vi "Timing_DAQ.vi"() -> ()   [LabVIEW 2022 SP3]
uses:
  <vilib>/DAQmx/read.llb/DAQmx Read (Analog 1D DBL NChan 1Samp).vi
  <vilib>/Utility/file.llb/Write Delimited Spreadsheet (string).vi
  <vilib>/DAQmx/configure/timing.llb/DAQmx Timing (Sample Clock).vi
  <vilib>/DAQmx/miscellaneous.llb/DAQmx Fill In Error Info.vi
  <vilib>/Utility/file.llb/Write Delimited Spreadsheet (DBL).vi
panel:
  in  "file path (dialog if empty)":path
  out "iterations":i32
  out "relative seconds":dbl format="%_19f"
  out "eLASPSED time":dbl
  out "data":dbl[](array[numeric]) format="%0.2f"
  out "Gauge":dbl(knob) scale=-11.0..10.0
  out "error out 2":errorcluster
  in  "stop":bool
  in  "rate":dbl=1000.0 format="%0.2f"
  in  "number of samples":i32=100
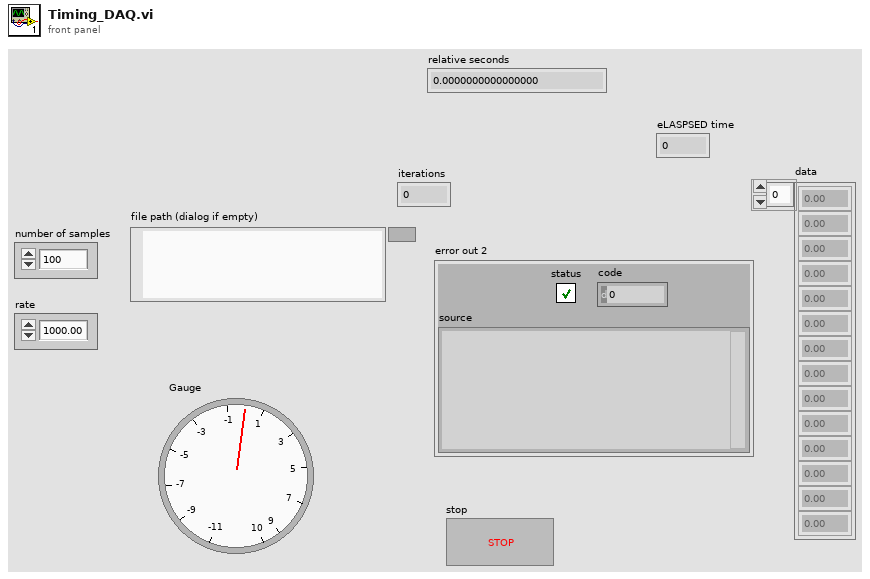
[diagram p1: front panel]
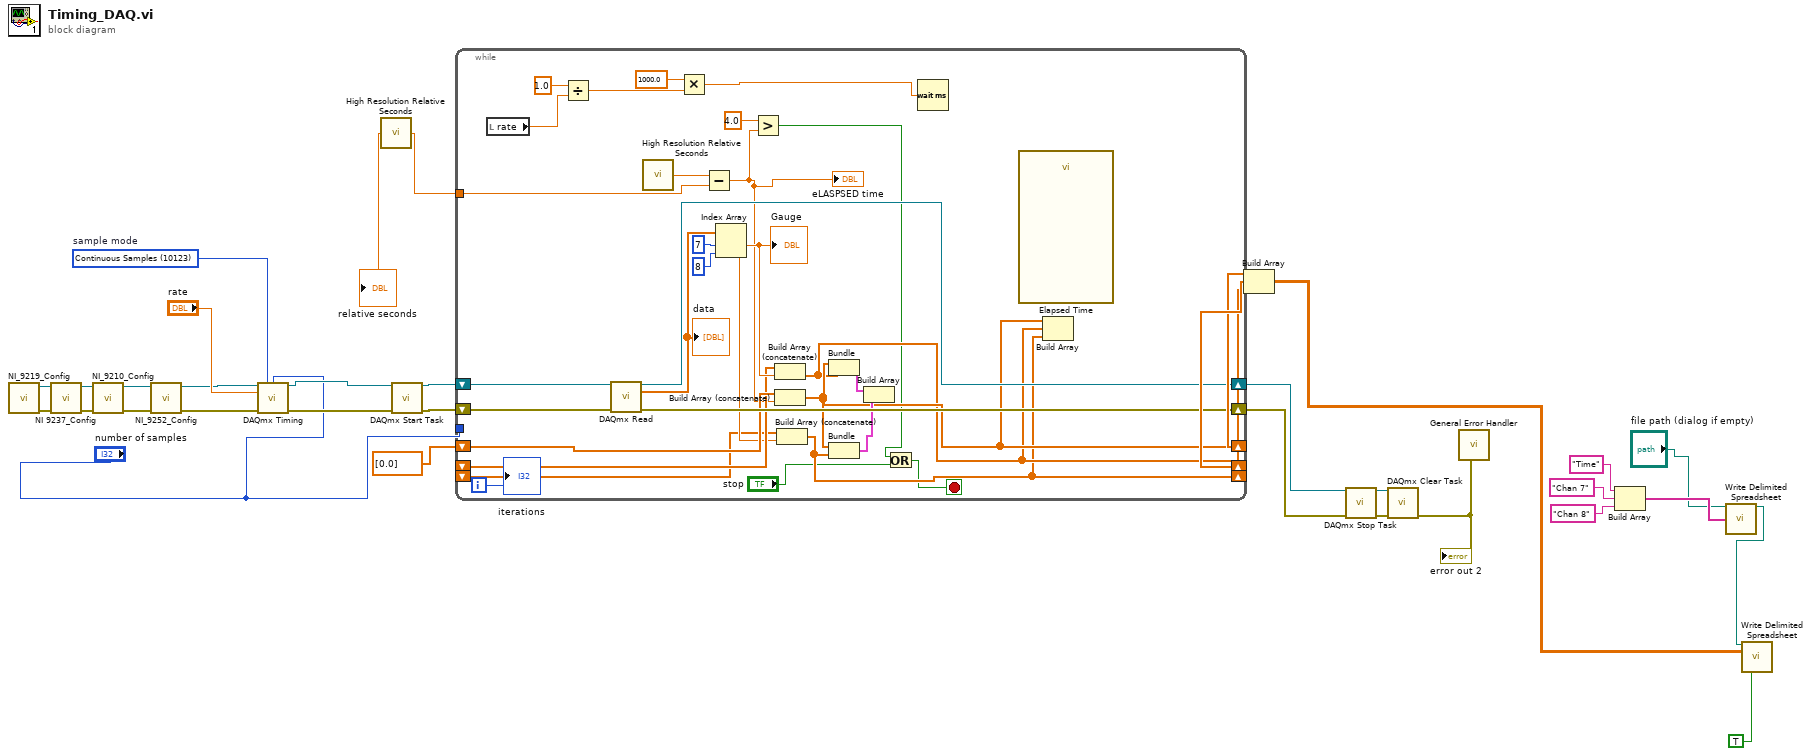
[diagram p0: block diagram]
diagram:
  w27 = 10123 items=["Finite Samples"=10178, "Continuous Samples"=10123, "Hardware Timed Single Point"=12522]  # sample mode
  n1 = call "NI_9219_Config.vi"() -> ("error out"=w28:errorcluster, "task out"=w33:refnum<k21>)  [unwired: 10 in]
  n2 = call "NI 9237_Config.vi"("error in"=w28, "task in"=w33) -> ("error out"=w31:errorcluster, "task out"=w32:refnum<k21>)  [unwired: 8 in]
  n3 = call "NI_9210_Config.vi"("error in"=w31, "task in"=w32) -> ("error out"=w29:errorcluster, "task out"=w30:refnum<k21>)  [unwired: 8 in]
  n4 = call "NI_9252_Config.vi"("error in"=w29, "task in"=w30) -> ("error out"=w24:errorcluster, "task out"=w25:refnum<k21>)  [unwired: 8 in]
  n5 = call-poly <vilib>:"DAQmx Timing.vi"("task/channels in"=w25, "sample mode"=w27, "samples per channel"="number of samples", "rate"="rate", "error in"=w24) -> ("task out"=w3:refnum<k21>, "error out"=w2:errorcluster)  [unwired: 9 in]
  n6 = call <vilib>:"High Resolution Relative Seconds.vi"() -> ("relative seconds"=w17:dbl)
  "relative seconds" <- w17
  n7 = call <vilib>:"DAQmx Start Task.vi"("task/channels in"=w3, "error in"=w2) -> ("task out"=w23:refnum<k21>, "error out"=w22:errorcluster)  [unwired: 12 in]
  n8 = while {
    shift-right: [w61] -> w18
    shift-left: w23 -> [w63]
    shift-right: [w60] -> w19
    shift-left: w22 -> [w62]
    tunnel: "number of samples" -> [_]
    tunnel: w17 -> [w57]
    shift-right: [w46] -> w13
    shift-left: dbl[] [0.0] -> [w56]
    shift-right: [w45] -> w15
    shift-left: _ -> [w53]
    shift-right: [w44] -> w14
    shift-left: _ -> [w50]
    i -> [w47]
    stop <- w42 stop-if-true
    n9 = local read "rate"() -> (w40:dbl)
    n10 = Divide(x=1.0, y=w40) -> (x/y=w39:dbl)
    n11 = call-poly <vilib>:"DAQmx Read.vi"("task/channels in"=w63, "error in"=w62) -> ("task out"=w61:refnum<k21>, "data"=w58:dbl[], "error out"=w60:errorcluster)  [unwired: 11 in]
    "data" <- w58
    n12 = call <vilib>:"High Resolution Relative Seconds.vi"() -> ("relative seconds"=w55:dbl)
    n13 = Multiply(x=1000.0, y=w39) -> (x*y=w37:dbl)
    n14 = Subtract(x=w55, y=w57) -> (x-y=w35:dbl)
    "eLASPSED time" <- w35
    n15 = Index Array(array=w58, index #1=7 ("index"), index #2=8 ("index")) -> (element #1=w54:dbl, element #2=w51:dbl)
    "Gauge" <- w54
    n16 = Greater?(x=4.0, y=w35) -> (0:w34:bool)
    n17 = Build Array (concatenate)(w53, w54) -> (w45:dbl[])
    n18 = Build Array (concatenate)(w56, w35) -> (w46:dbl[])
    n19 = Build Array (concatenate)(w50, w51) -> (w44:dbl[])
    n20 = Bundle(w46, w45) -> (w49:cluster{dbl[], dbl[]})  [unwired: 1 in]
    n21 = Bundle(w46, w44) -> (w48:cluster{dbl[], dbl[]})  [unwired: 1 in]
    n22 = Build Array(w49, w48) -> ()  [unwired: 1 out]
    n23 = Or(x=w34, y="stop") -> (x .or. y?=w42:bool)
    n24 = Wait (ms)(milliseconds to wait=w37) -> ()  [unwired: 1 out]
    n25 = call "Elapsed Time"() -> ()  [unwired: 12 in, 8 out]
    n26 = Build Array(w46, w45, w44) -> ()  [unwired: 1 out]
    "iterations" <- w47
  }
  n27 = Build Array(w13, w15, w14) -> (w10:dbl[][])
  n28 = call <vilib>:"DAQmx Stop Task.vi"("task/channels in"=w18, "error in"=w19) -> ("task out"=w21:refnum<k21>, "error out"=w20:errorcluster)  [unwired: 12 in]
  n29 = call <vilib>:"DAQmx Clear Task.vi"("task in"=w21, "error in"=w20) -> ("error out"=w16:errorcluster)  [unwired: 13 in]
  "error out 2" <- w16
  n30 = call <vilib>:"General Error Handler.vi"("error in (no error)"=w16) -> ()  [unwired: 10 in, 5 out]
  n31 = Build Array("Time", "Chan 7", "Chan 8") -> (w11:string[])
  n32 = call-poly <vilib>:"Write Delimited Spreadsheet.vi"("file path (dialog if empty)"="file path (dialog if empty)", "1D data"=w11) -> ("new file path (Not A Path if cancelled)"=w12:path)  [unwired: 12 in, 1 out]
  n33 = call-poly <vilib>:"Write Delimited Spreadsheet.vi"("file path (dialog if empty)"=w12, "2D data"=w10, "transpose? (no:F)"=TRUE) -> ()  [unwired: 11 in, 2 out]
